vi "tip-down-trigger.vi"(7 "TOL":fxp<+/-,16,5>, 8 "Vo":fxp<+/-,16,5>, 11 "e(k)":fxp<+/-,16,5>) -> (2 "trigger":bool)   [LabVIEW 2015, in "libimaging-cs.lvlib"]
doc: "When e(k) exceeds Vo +/- TOL,\nTRIGGER --> high."
uses:
  libimaging-cs.lvlib
panel:
  # "When e(k) exceeds Vo +/- TOL,\nTRIGGER --> high."
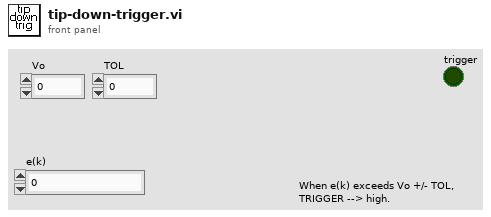
[diagram p1: front panel]
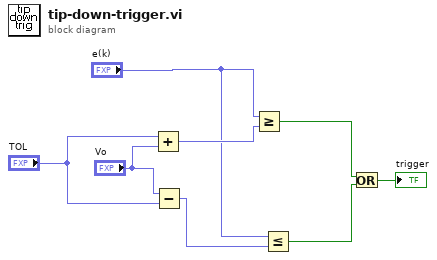
[diagram p0: block diagram]
diagram:
  n1 = Add(x="TOL", y="Vo") -> (x+y=w6:fxp<+/-,17,6>)
  n2 = Subtract(x="Vo", y="TOL") -> (x-y=w4:fxp<+/-,17,6>)
  n3 = Greater Or Equal?(x="e(k)", y=w6) -> (x >= y?=w3:bool)
  n4 = Less Or Equal?(x="e(k)", y=w4) -> (x <= y?=w2:bool)
  n5 = Or(x=w3, y=w2) -> (x .or. y?=→"trigger":bool)
